vi "Tag_InstrIO_Error_VIG.vi"(7 "Operation":enum16{"get data", "set data", "initialize"}(ring)=enum."set data", 8 "new element/subarray":errorcluster, 9 "Number of Sensors":i32, 10 "index":i32, 11 "tag_data_in":errorcluster[](array[cluster])) -> (2 "Error Status":bool[](array[boolean]), 3 "tag_data_out":errorcluster[](array[cluster]))   [LabVIEW 2018]
panel:
  # "---Error Indices---------\n0 -->DAQmx 6211\n1--->Agilent\n2-->Temp \n3--->FEM-03"
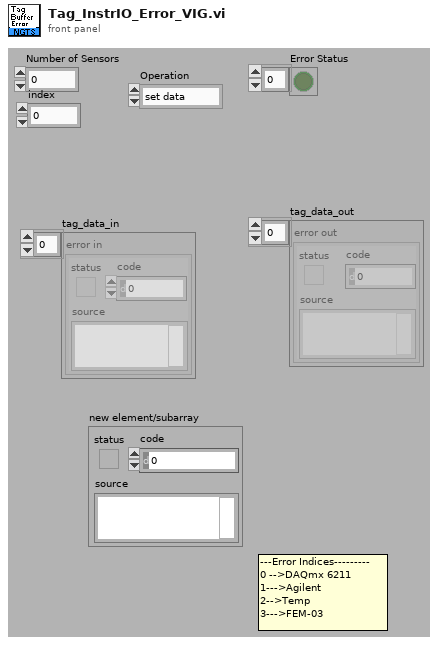
[diagram p1: front panel]
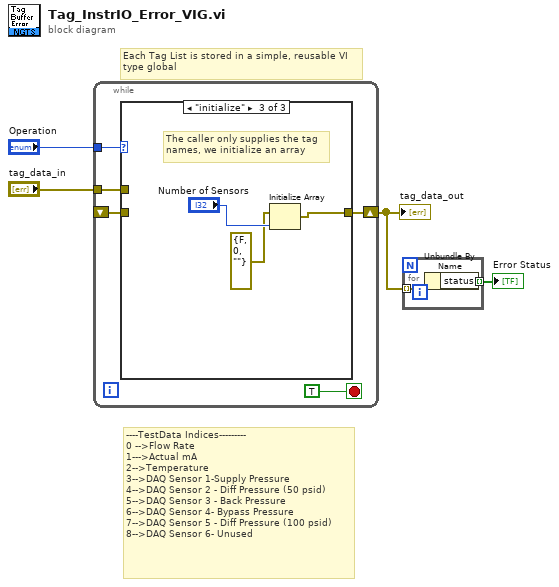
[diagram p0: block diagram]
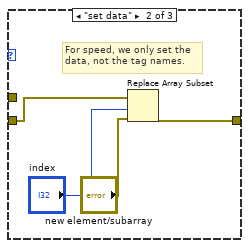
[diagram p3: hidden frame]
diagram:
  # "----TestData Indices---------\n0 -->Flow Rate\n1--->Actual mA \n2-->Temperature\n3-->DAQ Sensor 1-Supply Pressure\n4-->DAQ Sensor 2 - Diff Pressure (50 psid)\n5-->DAQ Sensor 3 - Back Pressure\n6-->DAQ Sensor 4- Bypass Pressure\n7-->DAQ Sensor 5 - Diff Pressure (100 psid)\n8-->DAQ Sensor 6- Unused"
  # "Each Tag List is stored in a simple, reusable VI\ntype global"
  n1 = while {
    tunnel: "Operation" -> [w9]
    shift-right: [w7] -> w2
    shift-left: _ -> [w5]
    tunnel: "tag_data_in" -> [w6]
    stop <- TRUE stop-if-true
    n2 = case shown="\"initialize\"" w9 {
      tunnel: [w10 w14 w16] -> w7
      tunnel: w6 -> [_ _ _]
      tunnel: w5 -> [w10 w11 _]
      frame "get data", Default {
      }
      frame "set data" {
        # "For speed, we only set the\ndata, not the tag names."
        n3 = Replace Array Subset(array=w11, new element="new element/subarray", index="index") -> (w14:errorcluster[])
      }
      frame "initialize" {
        # "The caller only supplies the tag\nnames, we initialize an array"
        n4 = Initialize Array(errorcluster {"status"=FALSE, "code"=0, "source"=""} ("new element/subarray"), "Number of Sensors") -> (w16:errorcluster[])
      }
    }
  }
  "tag_data_out" <- w2
  n5 = for {
    tunnel: w2 -> [w19] mode=indexing
    tunnel: [w18] -> w1 mode=indexing
    n6 = Unbundle By Name(w19) -> ("status"=w18:bool)
  }
  "Error Status" <- w1
